vi "Error Decoder.vi"(4 "Error In":errorcluster, 7 "StdOut Return":string) -> (0 "error out":errorcluster, 3 "Other Messages":string[](array[string]))   [LabVIEW 2015, in "StdOut Operations.lvlib"]
uses:
  StdOut Operations.lvlib
  Data Manipulation/Data Manipulation.lvlib
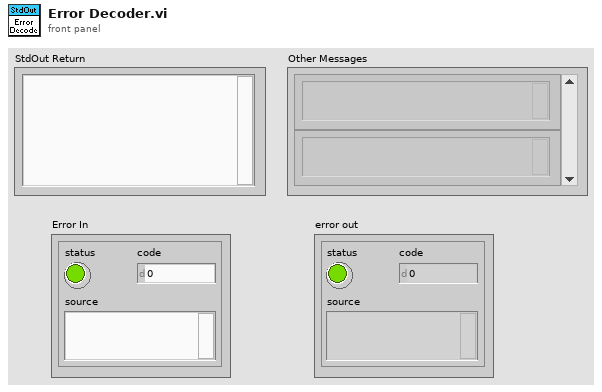
[diagram p1: front panel]
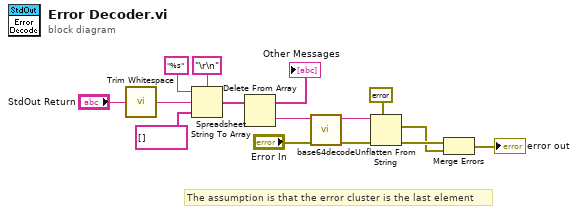
[diagram p0: block diagram]
diagram:
  # "The assumption is that the error cluster is the last element"
  n1 = call <vilib>:"Trim Whitespace.vi"("string"="StdOut Return") -> ("trimmed string"=w4:string)  [unwired: 1 in]
  n2 = Spreadsheet String To Array(delimiter (Tab)="\r\n" ("format string"), format string="%s", spreadsheet string=w4, array type (2D Dbl)=string[] []) -> (array=w6:string[])
  n3 = Delete From Array(array=w6) -> (deleted portion=w13:string, array with subset deleted=→"Other Messages":string[])  [unwired: 2 in]
  n4 = call "base64decode.vi"("Error In"="Error In", "string in (base64-encoded)"=w13) -> ("Error Out"=w11:errorcluster, "string out (decoded)"=w12:string)  [unwired: 4 in]
  n5 = Unflatten From String(type=errorcluster {"status"=FALSE, "code"=0, "source"=""}, binary string=w12, error in (no error)=w11) -> (value=w1:errorcluster, error out=w15:errorcluster)  [unwired: 2 in, 1 out]
  n6 = Merge Errors(w15, w1) -> (→"error out":errorcluster)
